vi "New File.vi"(8 "error in (no error)":errorcluster, 11 "Excel Interface in":refnum<class "Excel Interface.lvclass">) -> (0 "error out":errorcluster, 3 "Excel Interface out":refnum<class "Excel Interface.lvclass">)   [LabVIEW 2016, in "Excel Interface.lvclass"]
uses:
  Excel Interface.lvclass
  Excel Interface.lvclass/Excel Interface.ctl
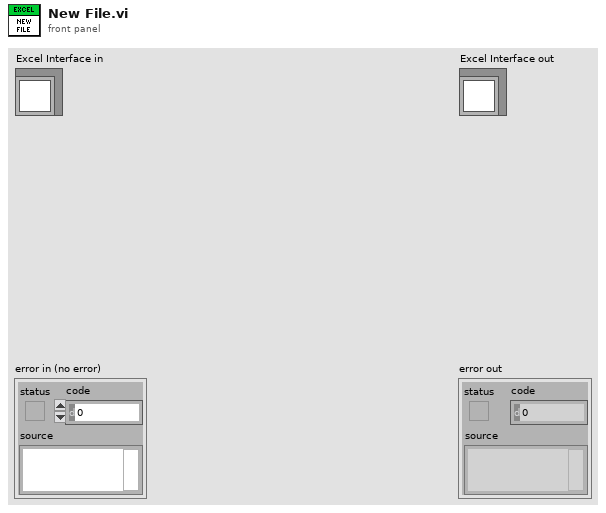
[diagram p1: front panel]
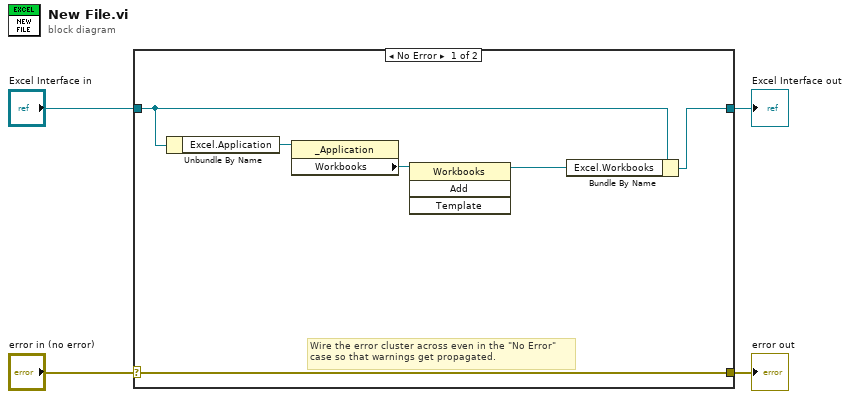
[diagram p0: block diagram]
diagram:
  n1 = case shown="No Error" "error in (no error)" {
    selector: "error in (no error)" -> [w10 w12]
    tunnel: [w10 w12] -> w3
    tunnel: [w6 w11] -> w1
    tunnel: "Excel Interface in" -> [w7 w11]
    frame No Error {
      # "Wire the error cluster across even in the \"No Error\"\ncase so that warnings get propagated."
      n2 = Unbundle By Name(w7) -> ("Excel.Application"=w9:refnum<k7>)
      n3 = property class="_Application"(reference=w9) -> ("Workbooks"=w8:refnum<k7>)  [unwired: 1 in, 2 out]
      n4 = invoke class="Workbooks" method="Add"(reference=w8) -> (reference out=w5:refnum<k7>)  [unwired: 3 in, 3 out]
      n5 = Bundle By Name(cluster=w7, "Excel.Workbooks"=w5) -> (w6:refnum<class "Excel Interface.lvclass">)
    }
    frame Error {
    }
  }
  "error out" <- w3
  "Excel Interface out" <- w1
